vi "VAttrbutesToData.vi"(7 "Prototype":variant, 8 "error in (no error)":errorcluster, 11 "VAttributes":variant) -> (0 "error out":errorcluster, 3 "data":variant)   [LabVIEW 2019]
uses:
  <userlib>/_OpenG.lib/error/error.llb/Build Error Cluster__ogtk.vi
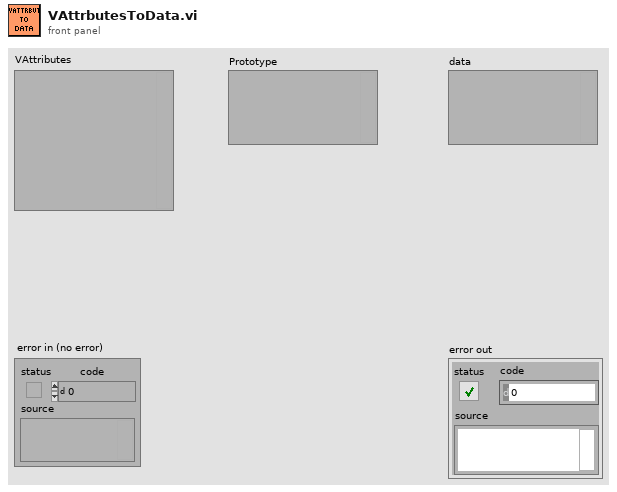
[diagram p1: front panel]
types:
  T1 = typedef "Type Descriptor Enumeration__ogtk.ctl" = enum8{"<Null>", "I8", "I16", "I32", "I64", "U8", "U16", "U32", "U64", "SGL", "DBL", "EXT", "CSG", "CDB", "CXT", "0x0F", "0x10", "0x11", "0x12", "0x13", "0x14", "Enum U8", "Enum U16", "Enum U32", "Enum U64", "SGL PQ", "DBL PQ", "EXT PQ", "CSG PQ", "CDB PQ", "CXT PQ", "0x1F", "0x20", "Boolean", "0x22", "0x23", "0x24", "0x25", "0x26", "0x27", "0x28", "0x29", "0x2A", "0x2B", "0x2C", "0x2D", "0x2E", "0x2F", "String", "0x31", "Path", "Pict", "0x34", "0x35", "0x36", "DAQ", "0x38", "0x39", "0x3A", "0x3B", "0x3C", "0x3D", "0x3E", "0x3F", "Array", "0x41", "0x42", "0x43", "0x44", "0x45", "0x46", "0x47", "0x48", "0x49", "0x4A", "0x4B", "0x4C", "0x4D", "0x4E", "0x4F", "Cluster", "0x51", "0x52", "Variant", "Waveform", "0x55", "0x56", "0x57", "0x58", "0x59", "0x5A", "0x5B", "0x5C", "0x5D", "0x5E", "0x5F", "0x60", "0x61", "0x62", "0x63", "0x64", "0x65", "0x66", "0x67", "0x68", "0x69", "0x6A", "0x6B", "0x6C", "0x6D", "0x6E", "0x6F", "Refnum"}
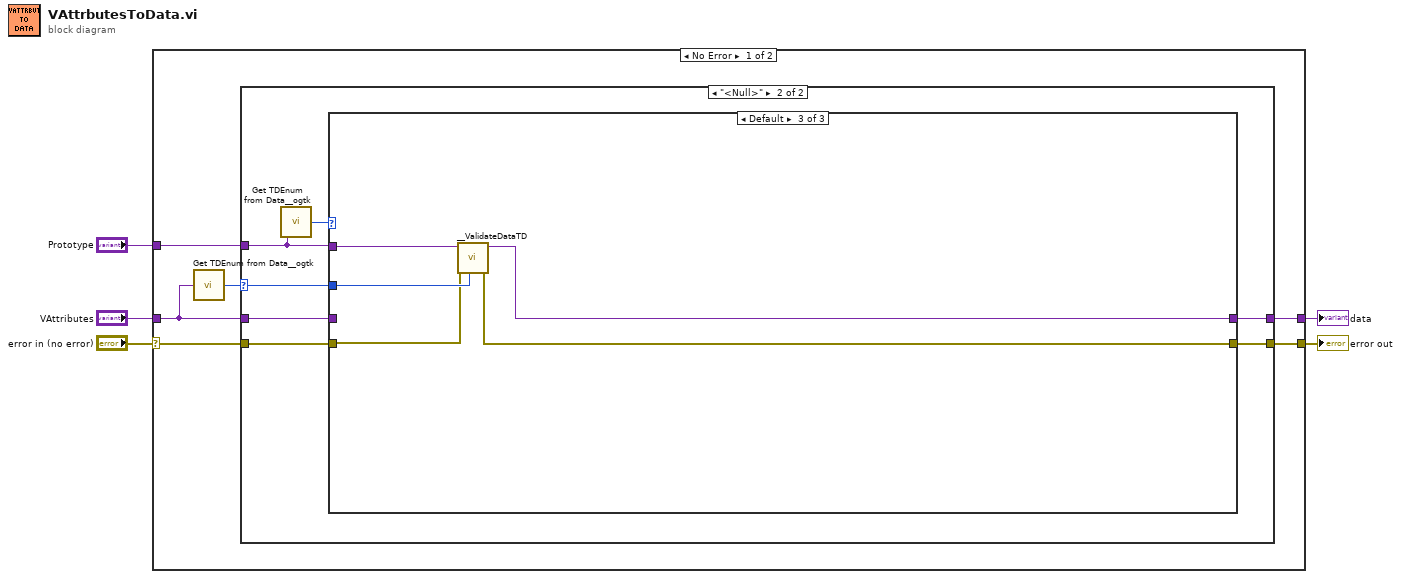
[diagram p0: block diagram]
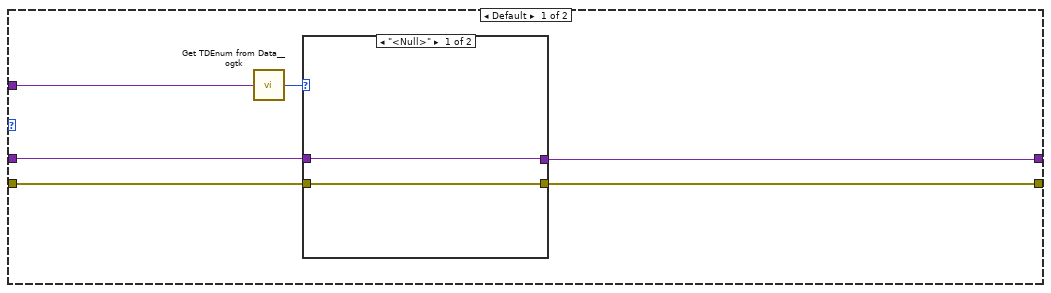
[diagram p2: hidden frame]
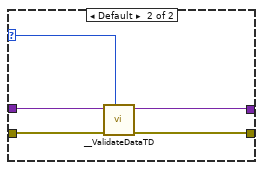
[diagram p3: hidden frame]
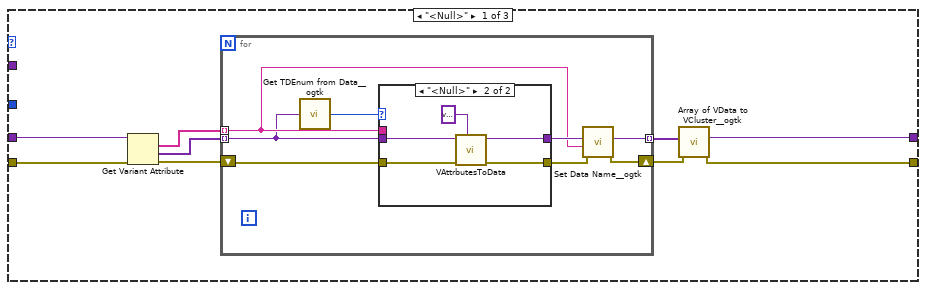
[diagram p4: hidden frame]
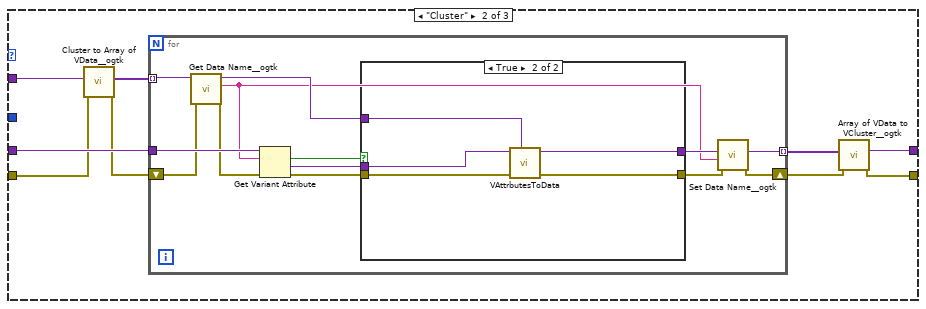
[diagram p6: hidden frame]
diagram:
  n1 = case shown="No Error" "error in (no error)" {
    selector: "error in (no error)" -> [w9 w90]
    tunnel: [w11 _] -> w5
    tunnel: [w10 w90] -> w4
    tunnel: "VAttributes" -> [w8 _]
    tunnel: "Prototype" -> [w6 _]
    frame No Error {
      n2 = call <userlib>:"Get TDEnum from Data__ogtk.vi"("Data"=w8) -> ("Type Descriptor Enumeration"=w7:T1)  [unwired: 4 in]
      n3 = case shown="\"<Null>\"" w7 {
        selector: w7 -> [_ w25]
        tunnel: [w15 w31] -> w11
        tunnel: [w17 w30] -> w10
        tunnel: w9 -> [w13 w29]
        tunnel: w6 -> [w16 w27]
        tunnel: w8 -> [w14 w26]
        frame Default {
          n4 = call <userlib>:"Get TDEnum from Data__ogtk.vi"("Data"=w16) -> ("Type Descriptor Enumeration"=w12:T1)  [unwired: 4 in]
          n5 = case shown="\"<Null>\"" w12 {
            selector: w12 -> [_ w22]
            tunnel: w13 -> [w18 w23]
            tunnel: [w18 w21] -> w17
            tunnel: w14 -> [w19 w24]
            tunnel: [w19 w20] -> w15
            frame "<Null>" {
            }
            frame Default {
              n6 = call "__ValidateDataTD.vi"("Expected TD"=w22, "error in (no error)"=w23, "Data"=w24) -> ("error out"=w21:errorcluster, "Data(dup)"=w20:variant)  [unwired: 7 in]
            }
          }
        }
        frame "<Null>" {
          n7 = call <userlib>:"Get TDEnum from Data__ogtk.vi"("Data"=w27) -> ("Type Descriptor Enumeration"=w28:T1)  [unwired: 4 in]
          n8 = case shown="Default" w28 {
            tunnel: w26 -> [w37 w64 _]
            tunnel: [w40 w63 w88] -> w31
            tunnel: [w39 w62 w85] -> w30
            tunnel: w29 -> [w38 w58 w86]
            tunnel: w27 -> [_ w59 w89]
            tunnel: w25 -> [_ _ w87]
            frame "<Null>" {
              n9 = Get Variant Attribute(Variant=w37, error in=w38) -> (names=w35:string[], values=w36:variant[], error out=w33:errorcluster)  [unwired: 2 in, 1 out]
              n10 = for {
                tunnel: w36 -> [w42] mode=indexing
                tunnel: w35 -> [w45] mode=indexing
                tunnel: [w48] -> w34 mode=indexing
                shift-right: [w47] -> w32
                shift-left: w33 -> [w44]
                n11 = call <userlib>:"Get TDEnum from Data__ogtk.vi"("Data"=w42) -> ("Type Descriptor Enumeration"=w41:T1)  [unwired: 4 in]
                n12 = case shown="\"<Null>\"" w41 {
                  tunnel: w42 -> [w50 w55]
                  tunnel: [w50 w54] -> w46
                  tunnel: w45 -> [_ _]
                  tunnel: w44 -> [w49 w53]
                  tunnel: [w49 w52] -> w43
                  frame Default {
                  }
                  frame "<Null>" {
                    n13 = call "VAttrbutesToData.vi"("Prototype"=variant, "error in (no error)"=w53, "VAttributes"=w55) -> ("error out"=w52:errorcluster, "data"=w54:variant)  [unwired: 7 in]
                  }
                }
                n14 = call <userlib>:"Set Data Name__ogtk.vi"("error in (no error)"=w43, "Data Name"=w45, "Data"=w46) -> ("error out"=w47:errorcluster, "Renamed Data"=w48:variant)  [unwired: 7 in]
              }
              n15 = call <userlib>:"Array of VData to VCluster__ogtk.vi"("error in (no error)"=w32, "Array"=w34) -> ("error out"=w39:errorcluster, "VCluster"=w40:variant)  [unwired: 8 in]
            }
            frame "Cluster" {
              n16 = call <userlib>:"Cluster to Array of VData__ogtk.vi"("error in (no error)"=w58, "Cluster"=w59) -> ("error out"=w57:errorcluster, "Array of VData"=w56:variant[])  [unwired: 8 in]
              n17 = for {
                tunnel: w64 -> [w77]
                tunnel: [w76] -> w61 mode=indexing
                shift-right: [w74] -> w60
                shift-left: w57 -> [w67]
                tunnel: w56 -> [w71] mode=indexing
                n18 = call <userlib>:"Get Data Name__ogtk.vi"("error in (no error)"=w67, "Data"=w71) -> ("error out"=w66:errorcluster, "Data Name"=w65:string, "Data dup"=w69:variant)  [unwired: 7 in]
                n19 = Get Variant Attribute(Variant=w77, name=w65, error in=w66) -> (found=w70:bool, value=w68:variant, error out=w75:errorcluster)  [unwired: 1 in, 1 out]
                n20 = case shown="True" w70 {
                  tunnel: w75 -> [w78 w81]
                  tunnel: [w79 w82] -> w73
                  tunnel: [w78 w80] -> w72
                  tunnel: w69 -> [w79 w83]
                  tunnel: w68 -> [_ w84]
                  frame False {
                  }
                  frame True {
                    n21 = call "VAttrbutesToData.vi"("Prototype"=w83, "error in (no error)"=w81, "VAttributes"=w84) -> ("error out"=w80:errorcluster, "data"=w82:variant)  [unwired: 7 in]
                  }
                }
                n22 = call <userlib>:"Set Data Name__ogtk.vi"("error in (no error)"=w72, "Data Name"=w65, "Data"=w73) -> ("error out"=w74:errorcluster, "Renamed Data"=w76:variant)  [unwired: 7 in]
              }
              n23 = call <userlib>:"Array of VData to VCluster__ogtk.vi"("error in (no error)"=w60, "Array"=w61) -> ("error out"=w62:errorcluster, "VCluster"=w63:variant)  [unwired: 8 in]
            }
            frame Default {
              n24 = call "__ValidateDataTD.vi"("Expected TD"=w87, "error in (no error)"=w86, "Data"=w89) -> ("error out"=w85:errorcluster, "Data(dup)"=w88:variant)  [unwired: 7 in]
            }
          }
        }
      }
    }
    frame Error {
    }
  }
  "data" <- w5
  "error out" <- w4
